vi "niRFUtil LCAPI Copy 1D Array (4 DBL).vi"(0 "Source0 1D Array (DBL)":dbl[](array[numeric]) format="%.2f", 5 "Source1 1D Array (DBL)":dbl[](array[numeric]) format="%.2f", 7 "Source2 1D Array (DBL)":dbl[](array[numeric]) format="%.2f", 9 "Source3 1D Array (DBL)":dbl[](array[numeric]) format="%.2f", 11 "error in (no error)":errorcluster, 12 "Data Copy Descriptor":u64) -> (4 "Source0 Out":dbl[](array[numeric]) format="%.2f", 6 "Source1 Out":dbl[](array[numeric]) format="%.2f", 8 "Source2 Out":dbl[](array[numeric]) format="%.2f", 10 "Source3 Out":dbl[](array[numeric]) format="%.2f", 15 "error out":errorcluster)   [LabVIEW 2015, in "niRFUtil.lvlib"]
uses:
  niRFUtil.lvlib
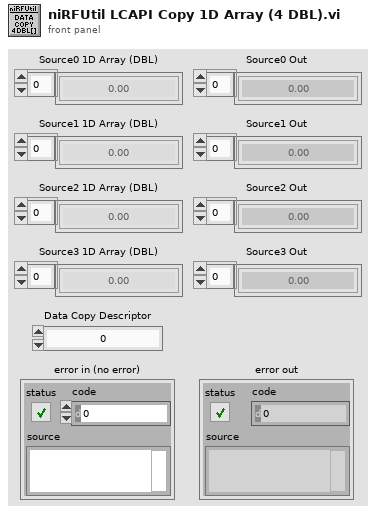
[diagram p1: front panel]
types:
  T1 = cluster{"status":bool, "return type":i32, "errorString":string}
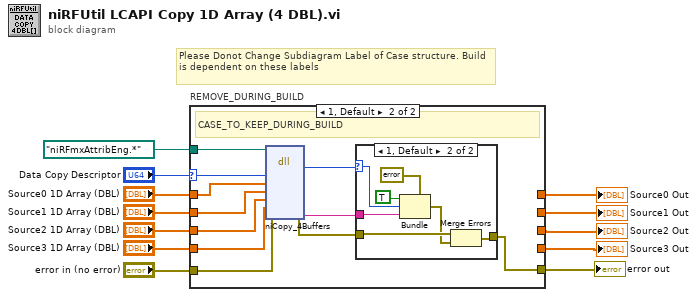
[diagram p0: block diagram]
diagram:
  # "Please Donot Change Subdiagram Label of Case structure. Build is dependent on these labels"
  n1 = case "REMOVE_DURING_BUILD" shown="1, Default" "Data Copy Descriptor" {
    selector: "Data Copy Descriptor" -> [_ w19]
    tunnel: [w13 w28] -> w12
    tunnel: "error in (no error)" -> [w13 w27]
    tunnel: "Source0 1D Array (DBL)" -> [w17 w26]
    tunnel: "Source1 1D Array (DBL)" -> [w16 w25]
    tunnel: "Source2 1D Array (DBL)" -> [w15 w24]
    tunnel: "Source3 1D Array (DBL)" -> [w14 w23]
    tunnel: [w17 _] -> w5
    tunnel: [w16 _] -> w4
    tunnel: [w15 _] -> w3
    tunnel: [w14 _] -> w2
    tunnel: path "niRFmxAttribEng.*" ("path in") -> [_ w18]
    frame 0 {
      # "Development"
    }
    frame 1, Default {
      # "CASE_TO_KEEP_DURING_BUILD"
      n2 = dll-call lib="niRFmxAttribEng.*" fn="niCopy_4Buffers"(path in=w18, error in=w27, "dataCopyDescriptor"=w19, "source0"=w26, "source1"=w25, "source2"=w24, "source3"=w23) -> (error out=w21:errorcluster, "return type"=w22:i32, "errorString"=w20:string)  [unwired: 7 in, 1 out]
      n3 = case shown="1, Default" w22 {
        selector: w22 -> [_ w34]
        tunnel: w20 -> [_ w35]
        tunnel: w21 -> [w29 w32]
        tunnel: [w29 w33] -> w28
        frame 0 {
        }
        frame 1, Default {
          n4 = Bundle(cluster=T1 {"status"=FALSE, "return type"=0, "errorString"=""}, "status"=TRUE, "return type"=w34, "errorString"=w35) -> (w31:T1)
          n5 = Merge Errors(w32, w31) -> (w33:errorcluster)
        }
      }
    }
  }
  "error out" <- w12
  "Source0 Out" <- w5
  "Source1 Out" <- w4
  "Source2 Out" <- w3
  "Source3 Out" <- w2
